vi "Save_Image.vi"(8 "error in (no error)":errorcluster, 9 "String":string, 10 "Scan Save Path":path, 11 "Refnum in":T1) -> (0 "error out":errorcluster)   [LabVIEW 2023, in "CameraLibrary.lvlib" / "Camera_Controller.lvlib"]
uses:
  Camera_Controller.lvlib
  <vilib>/vision/Image Controls.llb/IMAQ Image.ctl
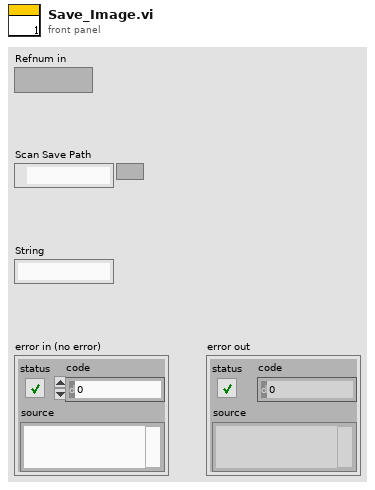
[diagram p1: front panel]
types:
  T1 = typedef "IMAQ Image.ctl" = refnum<image>
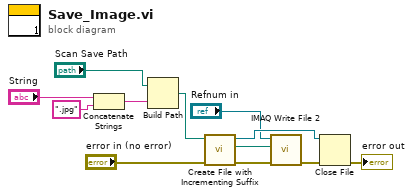
[diagram p0: block diagram]
diagram:
  n1 = Concatenate Strings("String", ".jpg" ("string")) -> (w2:string)
  n2 = Build Path(base path="Scan Save Path", name or relative path=w2) -> (appended path=w9:path)
  n3 = call <vilib>:"Create File with Incrementing Suffix.vi"("error in (no error)"="error in (no error)", "file path"=w9) -> ("error out"=w7:errorcluster, "actual path"=w8:path, "refnum out"=w10:refnum<file>)  [unwired: 7 in]
  n4 = call-poly "IMAQ Write File 2"("error in (no error)"=w7, "File Path"=w8, "Image"="Refnum in") -> ("error out"=w12:errorcluster)  [unwired: 7 in, 1 out]
  n5 = Close File(refnum=w10, error in=w12) -> (error out=→"error out":errorcluster)  [unwired: 1 out]
